vi "储运信息录入.vi"(1 "簇":T2 {"记录时间" format="%<%H:%M:%S\n%Y/%m/%d>T"}, 2 "connection reference":T1) -> (0 "负责人":i32)   [LabVIEW 2018]
uses:
  <vilib>/addons/database/Connection.llb/Conn ObjectReference.ctl
  <vilib>/addons/database/NI_Database_API.lvlib
panel:
  out "error out":errorcluster caption="错误输出"
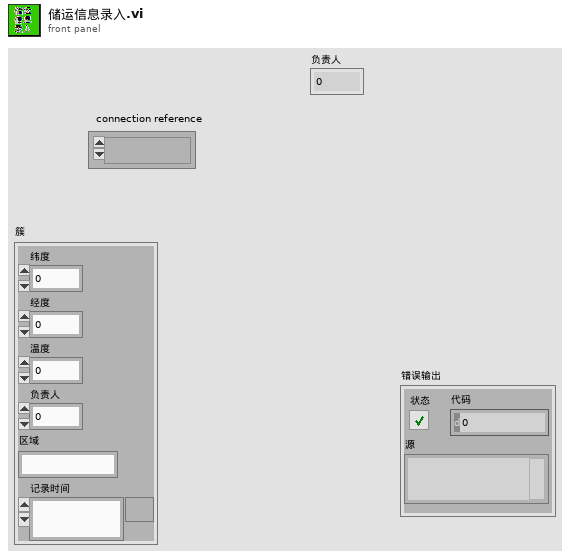
[diagram p1: front panel]
types:
  T1 = typedef "NI_Database_API.lvlib/Conn ObjectReference.ctl" = refnum<k1>
  T2 = typedef "储运信息.ctl" = cluster{"纬度":sgl, "经度":sgl, "温度":sgl, "负责人":i32, "区域":string, "记录时间":timestamp}
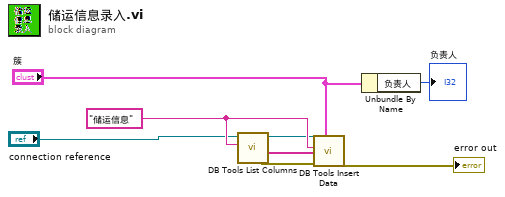
[diagram p0: block diagram]
diagram:
  w7 = "储运信息"
  n1 = call <vilib>:"DB Tools List Columns.vi"("table"=w7, "connection reference"="connection reference") -> ("error out"=w5:errorcluster, "columns"=w4:string[], "connection reference out"=w6:T1)  [unwired: 2 in, 1 out]
  n2 = call <vilib>:"DB Tools Insert Data.vi"("data"="簇", "error in (no error)"=w5, "columns"=w4, "table"=w7, "connection reference"=w6) -> ("error out"=→"error out":errorcluster)  [unwired: 5 in, 1 out]
  n3 = Unbundle By Name("簇") -> ("负责人"=→"负责人":i32)
